vi "VISA AMI430 Open.vi"(8 "error in (no error)":errorcluster, 10 "Timeout (ms)":u32=3000, 11 "VISA session":refnum<visa-resource-name>="TCPIP::146.201.232.88::7180::SOCKET") -> (0 "error out":errorcluster {"code" format="%.0x"}, 2 "Hello string":string, 3 "dup VISA Session":refnum<visa-resource-name>)   [LabVIEW 2019]
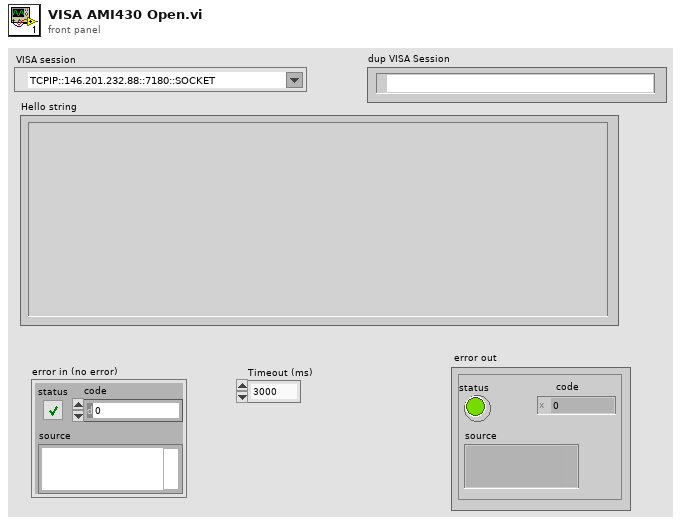
[diagram p1: front panel]
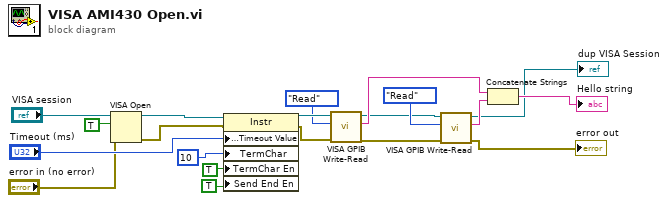
[diagram p0: block diagram]
diagram:
  n1 = VISA Open(duplicate session (F)=TRUE, error in (no error)="error in (no error)", VISA resource name="VISA session") -> (VISA resource name=w19:refnum<visa-resource-name>, error out=w17:errorcluster)  [unwired: 2 in]
  n2 = property class="Instr"(reference=w19, error in=w17, "General Settings:Timeout Value"="Timeout (ms)", "TermChar"=u8 10 ("Message Based Settings:Termination Character"), "TermChar En"=TRUE ("Message Based Settings:Termination Character Enable"), "Send End En"=TRUE ("Message Based Settings:Send End Enable")) -> (reference out=w15:refnum<visa-resource-name>, error out=w16:errorcluster)
  n3 = call "VISA GPIB Write-Read.vi"("error in (no error)"=w16, "Action"=enum16{"Write", "Read", "Write & Read"}."Read", "VISA resource name"=w15) -> ("error out"=w2:errorcluster, "String Returned"=w8:string, "dup VISA Session"=w5:refnum<visa-resource-name>)  [unwired: 5 in, 1 out]
  n4 = call "VISA GPIB Write-Read.vi"("error in (no error)"=w2, "Action"=enum16{"Write", "Read", "Write & Read"}."Read", "VISA resource name"=w5) -> ("error out"=→"error out":errorcluster, "String Returned"=w7:string, "dup VISA Session"=→"dup VISA Session":refnum<visa-resource-name>)  [unwired: 5 in, 1 out]
  n5 = Concatenate Strings(w8, w7) -> (→"Hello string":string)
